vi "Panel Resized.vi"(6 "Sizing Refnums 2":T2, 8 "error in (no error)":errorcluster, 9 "Origin":cluster{"H":i16, "V":i16}, 10 "NewBnds":T1, 11 "Size Constraints":cluster{"min tab width":i32, "w/h":dbl}) -> (0 "error out":errorcluster)   [LabVIEW 2016]
uses:
  <vilib>/Utility/miscctls.llb/LVRectTypeDef.ctl
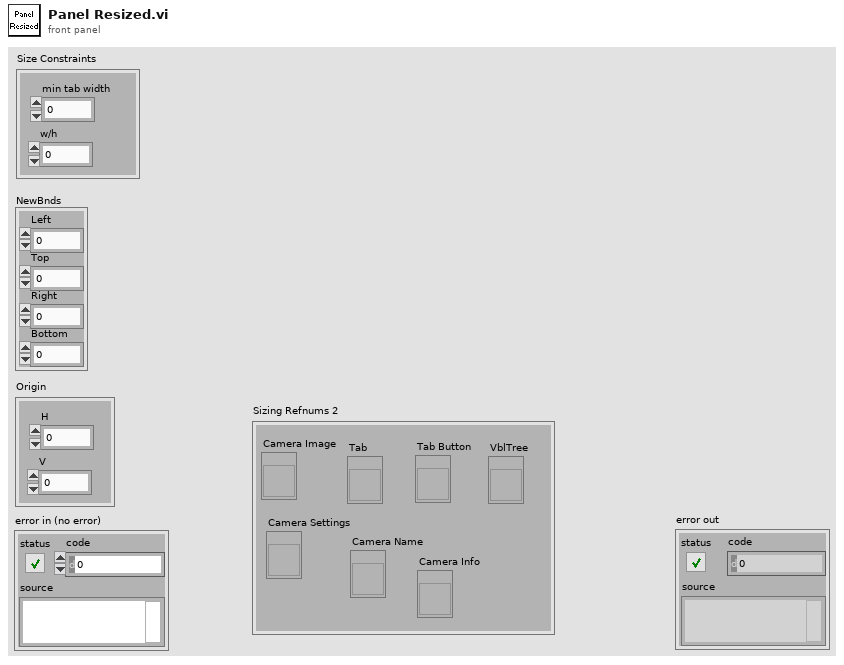
[diagram p1: front panel]
types:
  T1 = typedef "LVRectTypeDef.ctl" = cluster{"Left":i16, "Top":i16, "Right":i16, "Bottom":i16}
  T2 = cluster{"Camera Image":refnum<vi>, "Tab":refnum<vi>, "Tab Button":refnum<vi>, "VblTree":refnum<vi>, "Camera Settings":refnum<vi>, "Camera Name":refnum<vi>, "Camera Info":refnum<vi>}
  T3 = typedef "LVPositionTypeDef.ctl" = cluster{"Left":i32, "Top":i32}
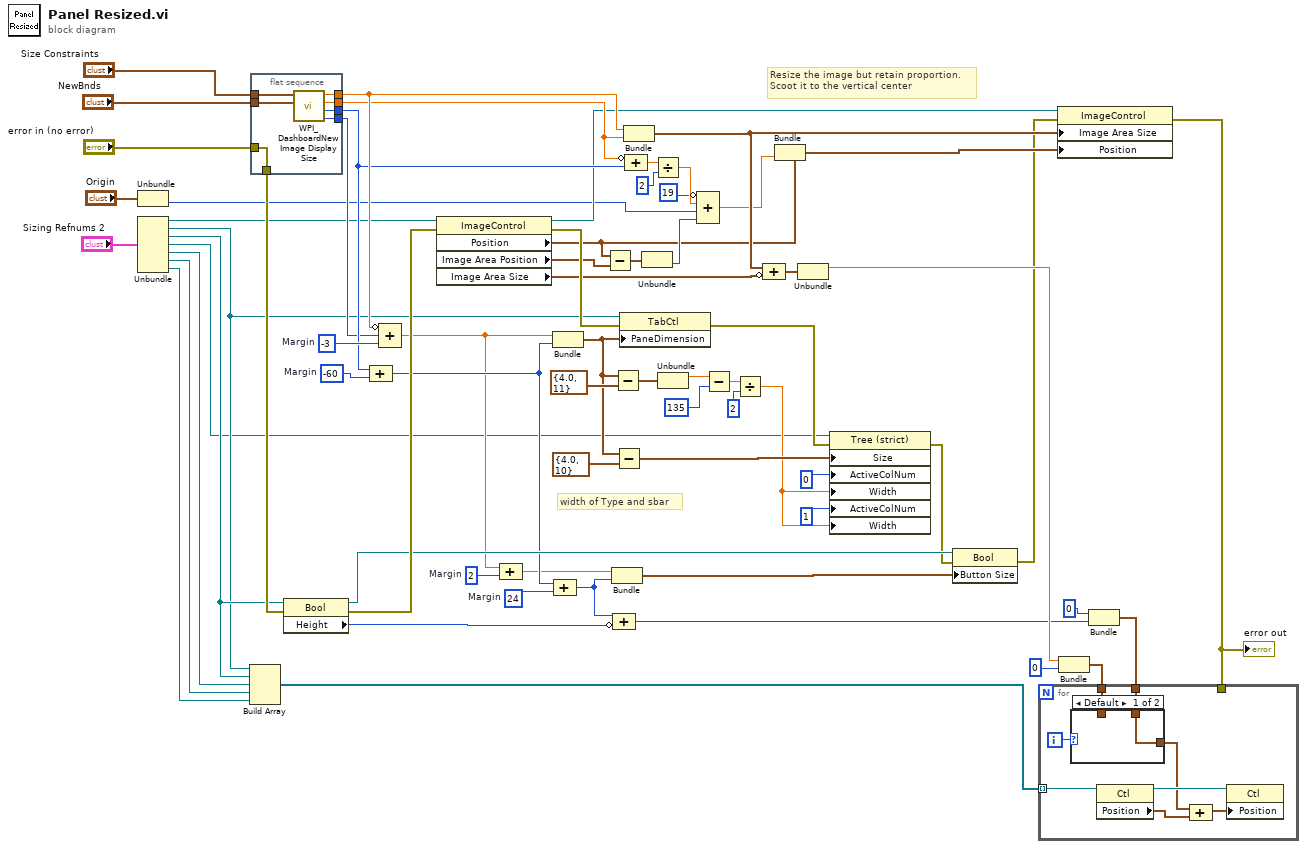
[diagram p0: block diagram]
diagram:
  w55 = 24  # Margin
  w53 = 2  # Margin
  w49 = -60  # Margin
  w59 = -3  # Margin
  # "width of Type and sbar"
  # "Resize the image but retain proportion.\nScoot it to the vertical center"
  n1 = Unbundle("Origin") -> ("V"=w30:i16)  [unwired: 1 out]
  n2 = Unbundle("Sizing Refnums 2") -> ("Camera Image"=w24:refnum<vi>, "Tab"=w25:refnum<vi>, "Tab Button"=w33:refnum<vi>, "VblTree"=w4:refnum<vi>, "Camera Settings"=w3:refnum<vi>, "Camera Name"=w2:refnum<vi>, "Camera Info"=w1:refnum<vi>)
  n3 = Build Array(w25, w33, w3, w2, w1) -> (w68:refnum<vi>[])
  n4 = flat-sequence {
    tunnel: "NewBnds" -> [w75]
    tunnel: "Size Constraints" -> [w74]
    tunnel: [w73] -> w48
    tunnel: [w72] -> w56
    tunnel: [w71] -> w57
    tunnel: [w70] -> w58
    tunnel: [w69] -> w67
    tunnel: "error in (no error)" -> [w69]
    frame #0 {
      n5 = call <vilib>:"WPI_DashboardNew Image Display Size.vi"("NewBnds"=w75, "Size Constraints"=w74) -> ("Window Width"=w73:i16, "Window Height"=w71:i16, "Height"=w72:dbl, "Width"=w70:dbl)  [unwired: 6 in]
    }
  }
  n6 = property class="Bool"(reference=w33, error in=w67) -> (reference out=w62:refnum<vi>, error out=w66:errorcluster, "Height"=w61:u32)
  n7 = Compound Arithmetic op=unknown(w57, w49) -> (w54:i32)
  n8 = Compound Arithmetic op=ADD(invert w58, w48, w59) -> (w52:dbl)
  n9 = property class="ImageControl"(reference=w24, error in=w66) -> (reference out=w41:refnum<vi>, error out=w65:errorcluster, "Position"=w40:T3, "Image Area Position"=w35:cluster{"Left":i32, "Top":i32}, "Image Area Size"=w46:cluster{"Width":u32, "Height":u32})
  n10 = Compound Arithmetic op=ADD(w52, w53) -> (w51:dbl)
  n11 = Bundle(w52, w54) -> (w10:cluster{dbl, i32})  [unwired: 1 in]
  n12 = Compound Arithmetic op=ADD(w54, w55) -> (w60:i32)
  n13 = Subtract(x=w40, y=w35) -> (x-y=w42:T3)
  n14 = Bundle(w51, w60) -> (w50:cluster{dbl, i32})  [unwired: 1 in]
  n15 = Subtract(x=w10, y=cluster{dbl, i32} {4.0, 11}) -> (x-y=w18:cluster{dbl, i32})
  n16 = Compound Arithmetic op=ADD(w60, invert w61) -> (w9:u32)
  n17 = Subtract(x=w10, y=cluster{dbl, i32} {4.0, 10}) -> (x-y=w21:cluster{dbl, i32})
  n18 = property class="TabCtl"(reference=w25, error in=w65, "PaneDimension"=w10) -> (error out=w6:errorcluster)  [unwired: 1 out]
  n19 = Bundle("Width"=w58, "Height"=w56) -> (w44:cluster{"Width":dbl, "Height":dbl})  [unwired: 1 in]
  n20 = Compound Arithmetic op=ADD(invert w56, w57) -> (w36:dbl)
  n21 = Unbundle(w42) -> ("Top"=w43:i32)  [unwired: 1 out]
  n22 = Divide(x=w36, y=2) -> (x/y=w38:dbl)
  n23 = Unbundle(w18) -> (w17:dbl)  [unwired: 1 out]
  n24 = Compound Arithmetic op=ADD(invert 19, w38, w30, w43) -> (w39:dbl)
  n25 = Subtract(x=w17, y=135 ("Active Cell:Active Column Number")) -> (x-y=w14:dbl)
  n26 = Divide(x=w14, y=2 ("Active Cell:Active Column Number")) -> (x/y=w8:dbl)
  n27 = Compound Arithmetic op=ADD(w44, invert w46) -> (w47:cluster{"Width":dbl, "Height":dbl})
  n28 = Bundle(cluster=w40, "Top"=w39) -> (w45:T3)  [unwired: 1 in]
  n29 = Unbundle(w47) -> ("Width"=w63:dbl)  [unwired: 1 out]
  n30 = property class="Tree (strict)"(reference=w4, error in=w6, "Size"=w21, "ActiveColNum"=0 ("Active Cell:Active Column Number"), "Width"=w8, "ActiveColNum"=1 ("Active Cell:Active Column Number"), "Width"=w8) -> (error out=w20:errorcluster)  [unwired: 1 out]
  n31 = property class="Bool"(reference=w62, error in=w20, "Button Size"=w50) -> (error out=w5:errorcluster)  [unwired: 1 out]
  n32 = property class="ImageControl"(reference=w41, error in=w5, "Image Area Size"=w44, "Position"=w45) -> (error out=w29:errorcluster)  [unwired: 1 out]
  "error out" <- w29
  n33 = Bundle("Width"=w63, 0) -> (w34:cluster{"Width":dbl, i32})  [unwired: 1 in]
  n34 = Bundle(0, w9) -> (w11:cluster{i32, u32})  [unwired: 1 in]
  n35 = for {
    tunnel: w68 -> [w83] mode=indexing
    tunnel: w34 -> [w78]
    tunnel: w29 -> [_]
    tunnel: w11 -> [w77]
    i -> [w79]
    n36 = case shown="Default" w79 {
      tunnel: w78 -> [_ w85]
      tunnel: w77 -> [w84 _]
      tunnel: [w84 w85] -> w76
      frame Default {
      }
      frame 0, 1 {
      }
    }
    n37 = property class="Ctl"(reference=w83) -> (reference out=w82:refnum<vi>, "Position"=w81:T3)  [unwired: 1 in, 1 out]
    n38 = Compound Arithmetic op=ADD(w76, w81) -> (w80:cluster{dbl, u32})
    n39 = property class="Ctl"(reference=w82, "Position"=w80) -> ()  [unwired: 1 in, 2 out]
  }
